vi "Write Outbound URI.vi"(10 "Outbound URI":string, 11 "Connection in":refnum<class "Connection.lvclass">) -> (3 "Connection out":refnum<class "Connection.lvclass">)   [LabVIEW 2013, in "Connection_GOSPL.lvlib" / "Connection.lvclass"]
uses:
  Connection.lvclass
  Connection.lvclass/Connection.ctl
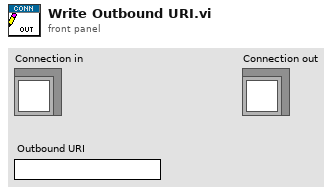
[diagram p1: front panel]
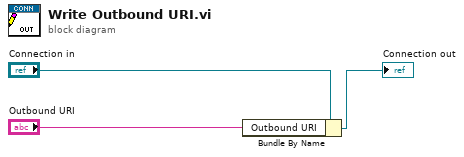
[diagram p0: block diagram]
diagram:
  n1 = Bundle By Name(cluster="Connection in", "Outbound URI"="Outbound URI") -> (→"Connection out":refnum<class "Connection.lvclass">)
